vi "Format Number Of Songs To String.vi"(1 "Number Of Songs":i32) -> (0 "Formatted":string)   [LabVIEW 2015, in "SongBrowserActor.lvlib" / "SongBrowserActor.lvclass"]
uses:
  SongBrowserActor.lvclass
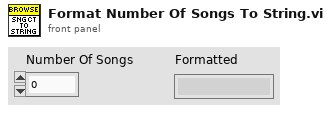
[diagram p1: front panel]
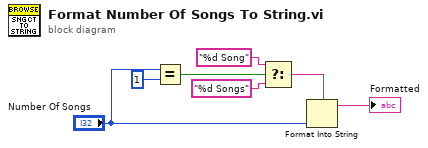
[diagram p0: block diagram]
diagram:
  n1 = Equal?(x="Number Of Songs", y=1) -> (x = y?=w4:bool)
  n2 = Select(t="%d Song" ("format string"), s=w4, f="%d Songs" ("format string")) -> (s? t:f=w3:string)
  n3 = Format Into String(format string=w3, "Number Of Songs") -> (resulting string=→"Formatted":string)  [unwired: 2 in, 1 out]
